vi "IPI_DrawRent.vi"() -> ()   [LabVIEW 2015]
panel:
  out "Image Out":T1(plugin-control)
  out "Image In":T1(plugin-control)
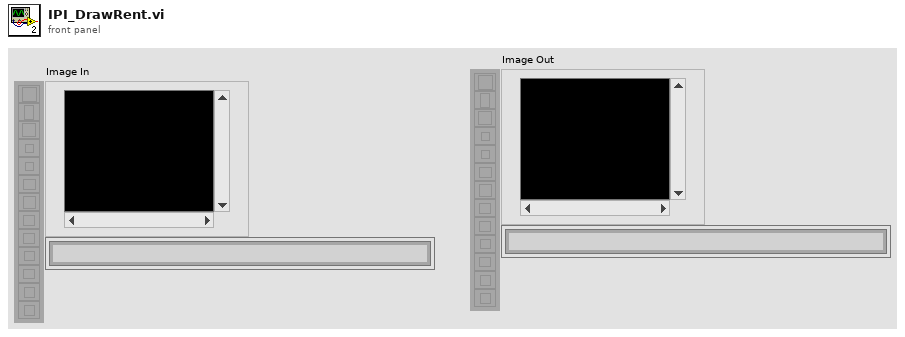
[diagram p1: front panel]
types:
  T1 = typedef "IMAQ Image.ctl" = refnum<image>
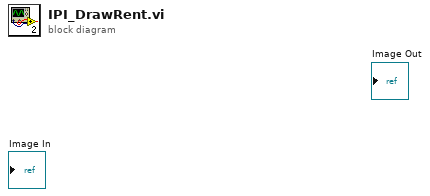
[diagram p0: block diagram]
diagram:
